vi "VI 서버 참조.vi"() -> ()   [LabVIEW 2014]
panel:
  out "데이터":dbl
  in  "클러스터":cluster{"숫자형":dbl, "불리언":bool, "문자열":string}
  in  "숫자형 2":dbl
  in  "숫자형":dbl
  in  "불리언":bool
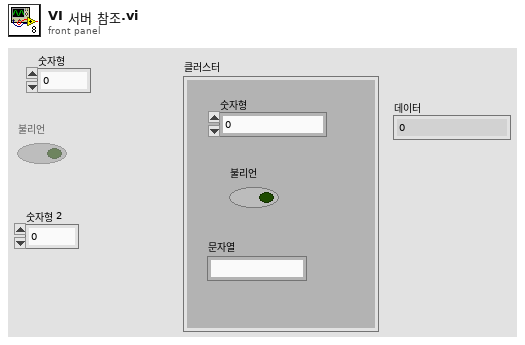
[diagram p1: front panel]
types:
  T1 = enum8{"Enabled", "Disabled", "Disabled and Grayed Out"}
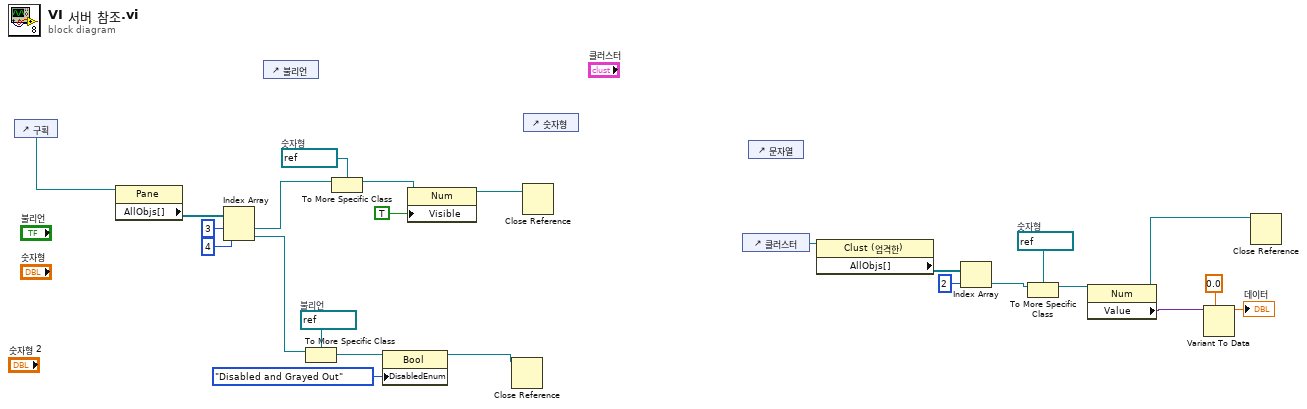
[diagram p0: block diagram]
diagram:
  w11 = refnum<vi> refnum  # 숫자형
  w21 = refnum<vi> refnum  # 숫자형
  w22 = refnum<vi> refnum  # 불리언
  n1 = control-ref of="구획"() -> (w24:refnum<vi>)
  n2 = property class="Pane"(reference=w24) -> ("AllObjs[]"=w23:refnum<vi>[])  [unwired: 1 in, 2 out]
  n3 = Index Array(array=w23, index #1=3 ("인덱스"), index #2=4 ("인덱스")) -> (element #1=w16:refnum<vi>, element #2=w15:refnum<vi>)
  n4 = control-ref of="불리언"() -> ()  [unwired: 1 out]
  n5 = To More Specific Class(target class=w22, reference=w15) -> (specific class reference=w20:refnum<vi>)  [unwired: 1 in, 1 out]
  n6 = To More Specific Class(target class=w21, reference=w16) -> (specific class reference=w19:refnum<vi>)  [unwired: 1 in, 1 out]
  n7 = property class="Bool"(reference=w20, "DisabledEnum"=T1."Disabled and Grayed Out" ("비활성화")) -> (reference out=w2:refnum<vi>)  [unwired: 1 in, 1 out]
  n8 = property class="Num"(reference=w19, "Visible"=TRUE ("보이기")) -> (reference out=w3:refnum<vi>)  [unwired: 1 in, 1 out]
  n9 = Close Reference(reference=w2) -> ()  [unwired: 1 in, 1 out]
  n10 = Close Reference(reference=w3) -> ()  [unwired: 1 in, 1 out]
  n11 = control-ref of="숫자형"() -> ()  [unwired: 1 out]
  n12 = control-ref of="클러스터"() -> (w14:refnum<vi>)
  n13 = control-ref of="문자열"() -> ()  [unwired: 1 out]
  n14 = property class="Clust (엄격한)"(reference=w14) -> ("AllObjs[]"=w13:refnum<vi>[])  [unwired: 1 in, 2 out]
  n15 = Index Array(array=w13, index=2 ("인덱스")) -> (element=w12:refnum<vi>)
  n16 = To More Specific Class(target class=w11, reference=w12) -> (specific class reference=w10:refnum<vi>)  [unwired: 1 in, 1 out]
  n17 = property class="Num"(reference=w10) -> (reference out=w1:refnum<vi>, "Value"=w6:variant)  [unwired: 1 in, 1 out]
  n18 = Variant To Data(type=0.0, Variant=w6) -> (data=→"데이터":dbl)  [unwired: 1 in, 1 out]
  n19 = Close Reference(reference=w1) -> ()  [unwired: 1 in, 1 out]
